vi "Write linkUUID.vi"(8 "error in (no error)":errorcluster, 10 "linkUUID":string, 11 "GrowableObjectFunction in":refnum<class "PropertyNode.lvclass">) -> (0 "error out":errorcluster, 3 "GrowableObjectFunction out":refnum<class "PropertyNode.lvclass">)   [LabVIEW 2025, in "PropertyNode.lvclass"]
uses:
  PropertyNode.lvclass
  PropertyNode.lvclass/PropertyNode.ctl
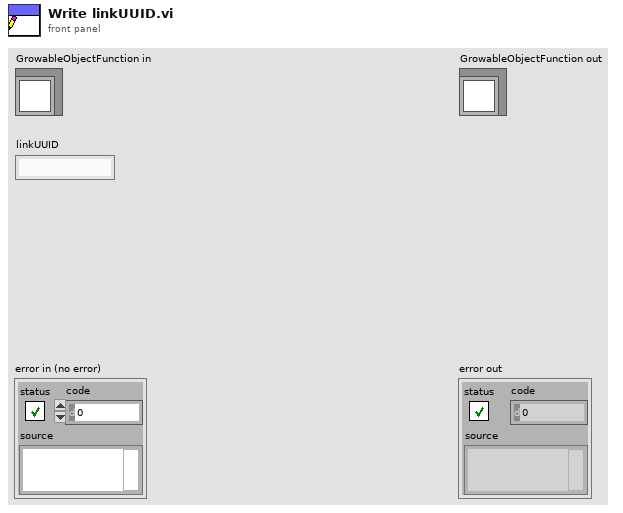
[diagram p1: front panel]
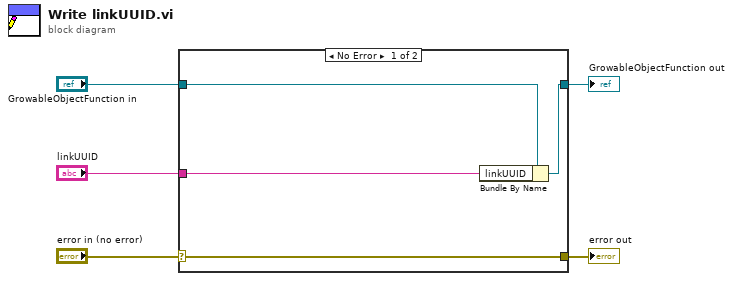
[diagram p0: block diagram]
diagram:
  n1 = case shown="No Error" "error in (no error)" {
    selector: "error in (no error)" -> [w9 w10]
    tunnel: [w9 w10] -> w4
    tunnel: [w7 w11] -> w2
    tunnel: "GrowableObjectFunction in" -> [w8 w11]
    tunnel: "linkUUID" -> [w6 _]
    frame No Error {
      n2 = Bundle By Name(cluster=w8, "linkUUID"=w6) -> (w7:refnum<class "PropertyNode.lvclass">)
    }
    frame Error {
    }
  }
  "error out" <- w4
  "GrowableObjectFunction out" <- w2
